vi "configuracion canales.vi"(4 "input cluster":T1) -> (0 "error out":errorcluster, 1 "task out":refnum<k21>)   [LabVIEW 2014]
uses:
  <vilib>/DAQmx/create/channels.llb/DAQmx Create Channel (AI-Voltage-Basic).vi
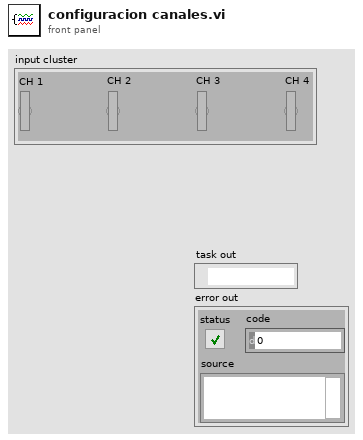
[diagram p1: front panel]
types:
  T1 = cluster{"CH 1":bool, "CH 2":bool, "CH 3":bool, "CH 4":bool}
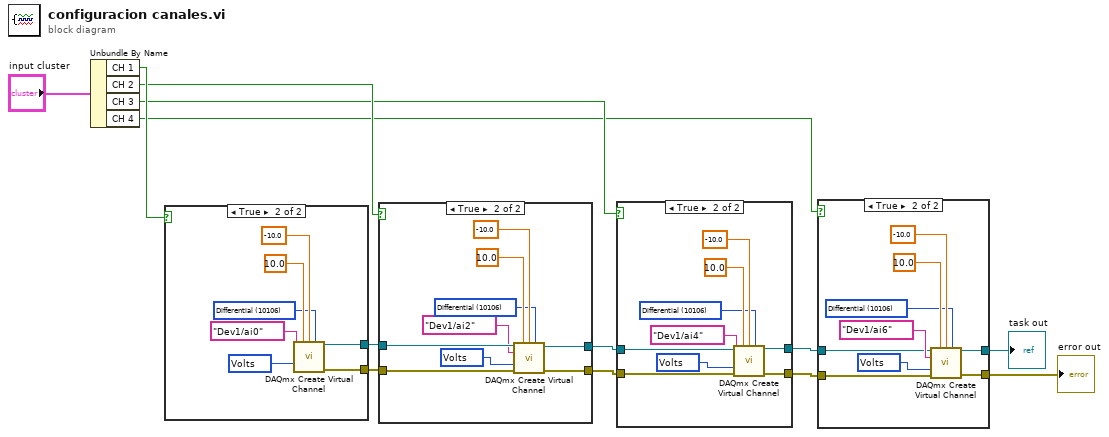
[diagram p0: block diagram]
diagram:
  n1 = Unbundle By Name("input cluster") -> ("CH 1"=w4:bool, "CH 2"=w3:bool, "CH 3"=w2:bool, "CH 4"=w1:bool)
  n2 = case shown="True" w4 {
    tunnel: [_ w20] -> w13
    tunnel: [_ w19] -> w12
    frame False {
    }
    frame True {
      w14 = 10106 items=["Default"=-1, "RSE"=10083, "NRSE"=10078, "Differential"=10106, "Pseudodifferential"=12529] ("input terminal configuration")
      w15 = 10348 items=["Volts"=10348, "From Custom Scale"=10065] ("units")
      n3 = call-poly <vilib>:"DAQmx Create Virtual Channel.vi"("maximum value"=10.0, "minimum value"=-10.0, "input terminal configuration"=w14, "physical channels"=tag "Dev1/ai0", "units"=w15) -> ("task out"=w20:refnum<k21>, "error out"=w19:errorcluster)  [unwired: 9 in]
    }
  }
  n4 = case shown="True" w3 {
    tunnel: w13 -> [w22 w31]
    tunnel: w12 -> [w21 w30]
    tunnel: [w22 w25] -> w9
    tunnel: [w21 w24] -> w8
    frame False {
    }
    frame True {
      w23 = 10106 items=["Default"=-1, "RSE"=10083, "NRSE"=10078, "Differential"=10106, "Pseudodifferential"=12529] ("input terminal configuration")
      w29 = 10348 items=["Volts"=10348, "From Custom Scale"=10065] ("units")
      n5 = call-poly <vilib>:"DAQmx Create Virtual Channel.vi"("task in"=w31, "maximum value"=10.0, "minimum value"=-10.0, "input terminal configuration"=w23, "physical channels"=tag "Dev1/ai2", "units"=w29, "error in"=w30) -> ("task out"=w25:refnum<k21>, "error out"=w24:errorcluster)  [unwired: 7 in]
    }
  }
  n6 = case shown="True" w2 {
    tunnel: [w32 w38] -> w11
    tunnel: [w33 w37] -> w10
    tunnel: w9 -> [w33 w36]
    tunnel: w8 -> [w32 w35]
    frame False {
    }
    frame True {
      w34 = 10106 items=["Default"=-1, "RSE"=10083, "NRSE"=10078, "Differential"=10106, "Pseudodifferential"=12529] ("input terminal configuration")
      w42 = 10348 items=["Volts"=10348, "From Custom Scale"=10065] ("units")
      n7 = call-poly <vilib>:"DAQmx Create Virtual Channel.vi"("task in"=w36, "maximum value"=10.0, "minimum value"=-10.0, "input terminal configuration"=w34, "physical channels"=tag "Dev1/ai4", "units"=w42, "error in"=w35) -> ("task out"=w37:refnum<k21>, "error out"=w38:errorcluster)  [unwired: 7 in]
    }
  }
  n8 = case shown="True" w1 {
    tunnel: w11 -> [w43 w49]
    tunnel: w10 -> [w44 w48]
    tunnel: [w44 w47] -> w7
    tunnel: [w43 w46] -> w6
    frame False {
    }
    frame True {
      w45 = 10106 items=["Default"=-1, "RSE"=10083, "NRSE"=10078, "Differential"=10106, "Pseudodifferential"=12529] ("input terminal configuration")
      w50 = 10348 items=["Volts"=10348, "From Custom Scale"=10065] ("units")
      n9 = call-poly <vilib>:"DAQmx Create Virtual Channel.vi"("task in"=w48, "maximum value"=10.0, "minimum value"=-10.0, "input terminal configuration"=w45, "physical channels"=tag "Dev1/ai6", "units"=w50, "error in"=w49) -> ("task out"=w47:refnum<k21>, "error out"=w46:errorcluster)  [unwired: 7 in]
    }
  }
  "task out" <- w7
  "error out" <- w6
